vi "Configure Constant Voltage.vi"(6 "Current Maximum (15.000)":dbl=15.0 min=0.0 max=725.0 step=1.0 format="%.3f", 8 "error in (no error)":errorcluster, 9 "Current Minimum (0)":dbl min=0.0 max=725.0 step=1.0 format="%.3f", 10 "CV Voltage (0.1)":dbl=0.1 min=0.0 max=500.0 step=1.0 format="%#.4g", 11 "VISA resource name":refnum<visa-resource-name>) -> (0 "error out":errorcluster, 3 "VISA resource name out":refnum<visa-resource-name>)   [LabVIEW 2018, in "BK Precision 8600 Series.lvlib"]
doc: "Configures the voltage and current max/min limit for constant voltage (CV) operation."
uses:
  <instrlib>/BK Precision 8600 Series/BK Precision 8600 Series.lvlib
panel:
  # "A"
  # "A"
  # "V"
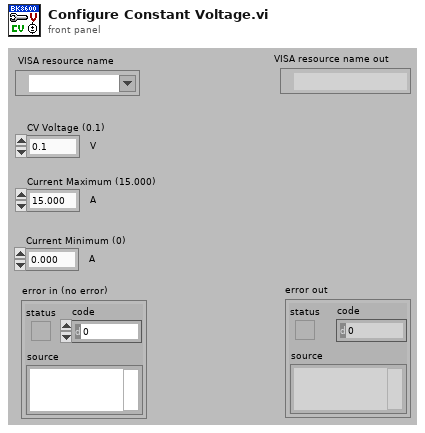
[diagram p1: front panel]
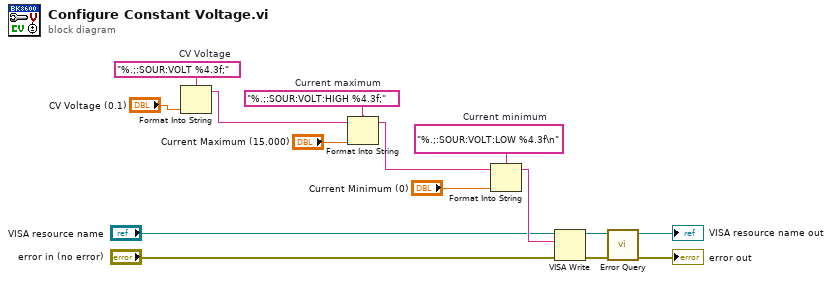
[diagram p0: block diagram]
diagram:
  w9 = "%.;:SOUR:VOLT:LOW %4.3f\n"  # Current minimum
  w3 = "%.;:SOUR:VOLT:HIGH %4.3f;"  # Current maximum
  w13 = "%.;:SOUR:VOLT %4.3f;"  # CV Voltage
  n1 = Format Into String(format string=w13, "CV Voltage (0.1)") -> (resulting string=w7:string)  [unwired: 2 in, 1 out]
  n2 = Format Into String(format string=w3, initial string=w7, "Current Maximum (15.000)") -> (resulting string=w8:string)  [unwired: 1 in, 1 out]
  n3 = Format Into String(format string=w9, initial string=w8, "Current Minimum (0)") -> (resulting string=w4:string)  [unwired: 1 in, 1 out]
  n4 = VISA Write(VISA resource name="VISA resource name", write buffer=w4, error in (no error)="error in (no error)") -> (VISA resource name out=w11:refnum<visa-resource-name>, error out=w12:errorcluster)  [unwired: 1 out]
  n5 = call <instrlib>:"Error Query.vi"("error in (no error)"=w12, "VISA resource name"=w11) -> ("error out"=→"error out":errorcluster, "VISA resource name out"=→"VISA resource name out":refnum<visa-resource-name>)  [unwired: 6 in, 2 out]
